vi "Show Networks.vi"(8 "error in (no error)":errorcluster) -> (0 "error out":errorcluster, 2 "SSID":string[](array[string]), 3 "Feedback":string)   [LabVIEW 2012]
doc: "Displays a list of wireless networks that are visible on the computer."
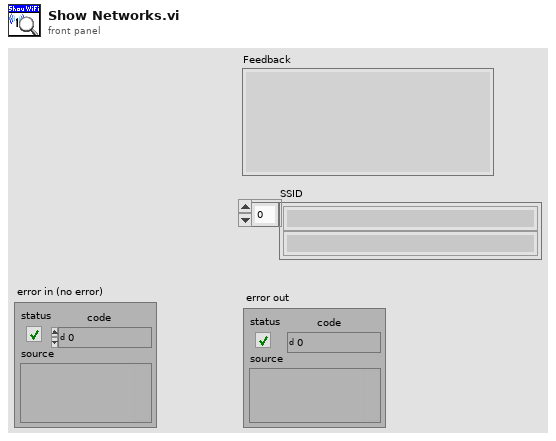
[diagram p1: front panel]
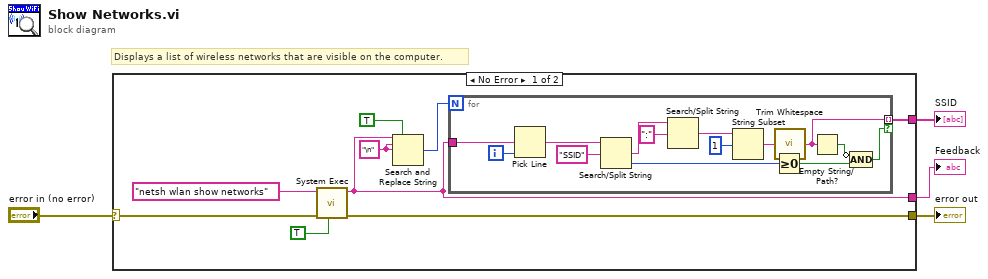
[diagram p0: block diagram]
diagram:
  # "Displays a list of wireless networks that are visible on the computer."
  n1 = case shown="No Error" "error in (no error)" {
    selector: "error in (no error)" -> [w7 w28]
    tunnel: [w8 w28] -> w4
    tunnel: [w6 _] -> w2
    tunnel: [w5 _] -> w1
    frame No Error {
      w11 = "\n" ("search string")
      n2 = call <vilib>:"System Exec.vi"("run minimized? (F)"=TRUE, "error in (no error)"=w7, "command line"="netsh wlan show networks") -> ("error out"=w8:errorcluster, "standard output"=w5:string)  [unwired: 5 in, 2 out]
      n3 = Search and Replace String(replace all?=TRUE ("replace all? (F)"), input string=w5, search string=w11, replace string=w11) -> (number of replacements=w9:i32)  [unwired: 4 in, 3 out]
      n4 = for {
        N: w9 -> [_]
        tunnel: w5 -> [w27]
        tunnel: [w16] -> w6 mode=indexing if=w15
        i -> [w26]
        n5 = Pick Line(multi-line string=w27, line index=w26) -> (output string=w25:string)  [unwired: 1 in]
        n6 = Search/Split String(string=w25, search string/char (-)="SSID") -> (match + rest of string=w23:string, offset of match=w21:i32)  [unwired: 1 in, 1 out]
        n7 = Search/Split String(string=w23, search string/char (-)=":") -> (match + rest of string=w19:string)  [unwired: 1 in, 2 out]
        n8 = String Subset(string=w19, offset (0)=1) -> (substring=w17:string)  [unwired: 1 in]
        n9 = Greater Or Equal To 0?(x=w21) -> (x >= 0?=w20:bool)
        n10 = call <vilib>:"Trim Whitespace.vi"("string"=w17) -> ("trimmed string"=w16:string)  [unwired: 1 in]
        n11 = Empty String/Path?(string/path=w16) -> (empty?=w14:bool)
        n12 = Compound Arithmetic op=AND(invert w14, w20) -> (w15:bool)
      }
    }
    frame Error {
    }
  }
  "error out" <- w4
  "SSID" <- w2
  "Feedback" <- w1
